vi "Commit.vi"(8 "error in (no error)":errorcluster, 11 "Initialize_card in":refnum<class "Initialize_card.lvclass">) -> (0 "error out":errorcluster, 3 "Initialize_card out":refnum<class "Initialize_card.lvclass">)   [LabVIEW 2015, in "Initialize_card.lvclass"]
uses:
  Initialize_card.lvclass
panel:
  out "Error String":string
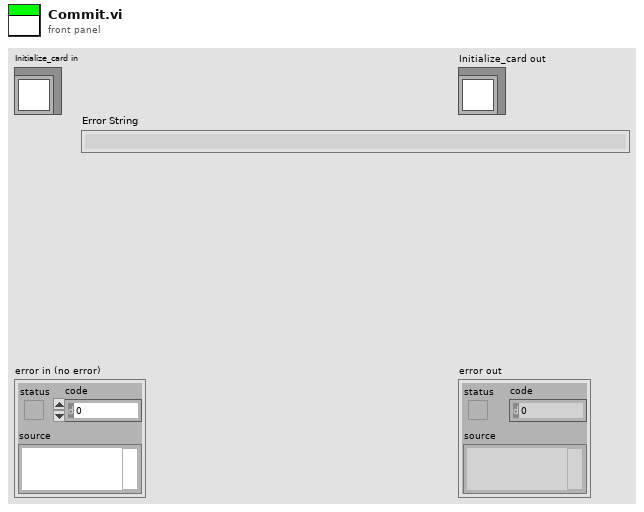
[diagram p1: front panel]
types:
  T1 = cluster{"Handle":u32, "Sample size":u32, "Resolution":i32, "Offset":i32, "Channels":u32, "Boards":u32}
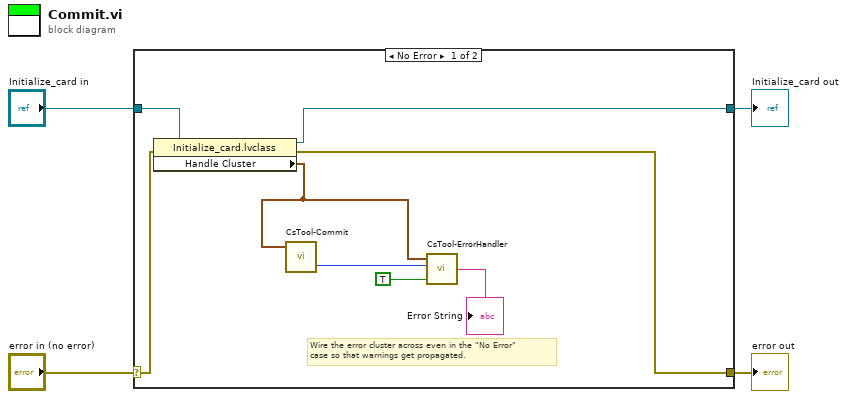
[diagram p0: block diagram]
diagram:
  n1 = case shown="No Error" "error in (no error)" {
    selector: "error in (no error)" -> [w8 w14]
    tunnel: [w7 w14] -> w3
    tunnel: [w9 w13] -> w1
    tunnel: "Initialize_card in" -> [w10 w13]
    frame No Error {
      # "Wire the error cluster across even in the \"No Error\"\ncase so that warnings get propagated."
      n2 = property class="Initialize_card.lvclass"(reference=w10, error in=w8) -> (reference out=w9:refnum<class "Initialize_card.lvclass">, error out=w7:errorcluster, "Handle Cluster"=w6:T1)
      n3 = call <userlib>:"CsTool-Commit.vi"("Handle Cluster"=w6) -> ("Error Code"=w12:i32)  [unwired: 2 in, 1 out]
      n4 = call <userlib>:"CsTool-ErrorHandler.vi"("StopOnError (true)"=TRUE, "Error Code"=w12, "Handle Cluster"=w6) -> ("Error String"=→"Error String":string)
    }
    frame Error {
    }
  }
  "error out" <- w3
  "Initialize_card out" <- w1
